vi "校准设置页.vi"() -> ()   [LabVIEW 2016, in "斯坦道CODMn.lvlib"]
uses:
  <vilib>/Analysis/6fits.llb/Curve Fitting Criteria.ctl
  <vilib>/Analysis/NI_AALPro.lvlib
  <vilib>/ptbypt/NI_PtbyPt.lvlib
panel:
  in  "读取公式":bool
  in  "历史数据导入":T1(radio)
  out "校准任务":bool
  in  "二次方程2":cluster{"K":dbl, "B":dbl, "x^2":dbl} {"x^2" format="%#.6g"; "K" format="%#.6g"; "B" format="%#.6g"}
  in  "公式切换阈值滴定数(0~9999)":dbl
  out "校准状态":T2(ring)
  out "模型刷新":bool
  in  "校准按钮":T1(radio)
  in  "校准导入":bool
  in  "曲线模型":T3={"标液浓度1"=0.0, "测量吸光度1"=0.0, "样品1启用"=FALSE, "标液浓度2"=0.0, "测量吸光度2"=0.0, "样品2启用"=FALSE, "标液浓度3"=0.0, "测量吸光度3"=0.0, "样品3启用"=FALSE, "标液浓度4"=0.0, "测量吸光度4"=0.0, "样品4启用"=FALSE, "标液浓度5"=0.0, "测量吸光度5"=0.0, "样品5启用"=FALSE, "模型"=enum."线性", "精度"=4.0, "XY图"=[], "拟合公式"="", "r^2"=0.0, "标样一校准时间"=timestamp(0 s since 1904-01-01), "标样二校准时间"=timestamp(0 s since 1904-01-01), "标样三校准时间"=timestamp(0 s since 1904-01-01), "标样四校准时间"=timestamp(0 s since 1904-01-01), "标样五校准时间"=timestamp(0 s since 1904-01-01), "二次方程"={"K"=0.0, "B"=0.0, "x^2"=0.0}, "标定时间"=timestamp(0 s since 1904-01-01), "拟合公式 2"="", "r^2 2"=0.0} {"r^2 2" format="%.7f"; "标定时间" format="%<%Y/%m/%d %H:%M:%S>T"; "二次方程"."x^2" format="%#.6g"; "二次方程"."K" format="%#.6g"; "二次方程"."B" format="%#.6g"; "标样五校准时间" format="%<%Y/%m/%d %H:%M:%S>T"; "标样四校准时间" format="%<%Y/%m/%d %H:%M:%S>T"; "标样三校准时间" format="%<%Y/%m/%d %H:%M:%S>T"; "标样二校准时间" format="%<%Y/%m/%d %H:%M:%S>T"; "标样一校准时间" format="%<%Y/%m/%d %H:%M:%S>T"; "r^2" format="%.7f"; "测量吸光度5" format="%#.6f"; "测量吸光度4" format="%#.6f"; "测量吸光度3" format="%#.6f"; "测量吸光度2" format="%#.6f"; "测量吸光度1" format="%#.6f"}
  in  "测量模式":T4(ring)
  in  "参数下拉列表":u16(ring) items=["CODMn"=21]
  in  "量程下拉列表":enum16{"低量程", "高量程"}(ring)
  # "校准时间"
  # "标液浓度"
  # "滴定数"
  # "标液一"
  # "标液二"
  # "标液三"
  # "零点"
  # "跨度"
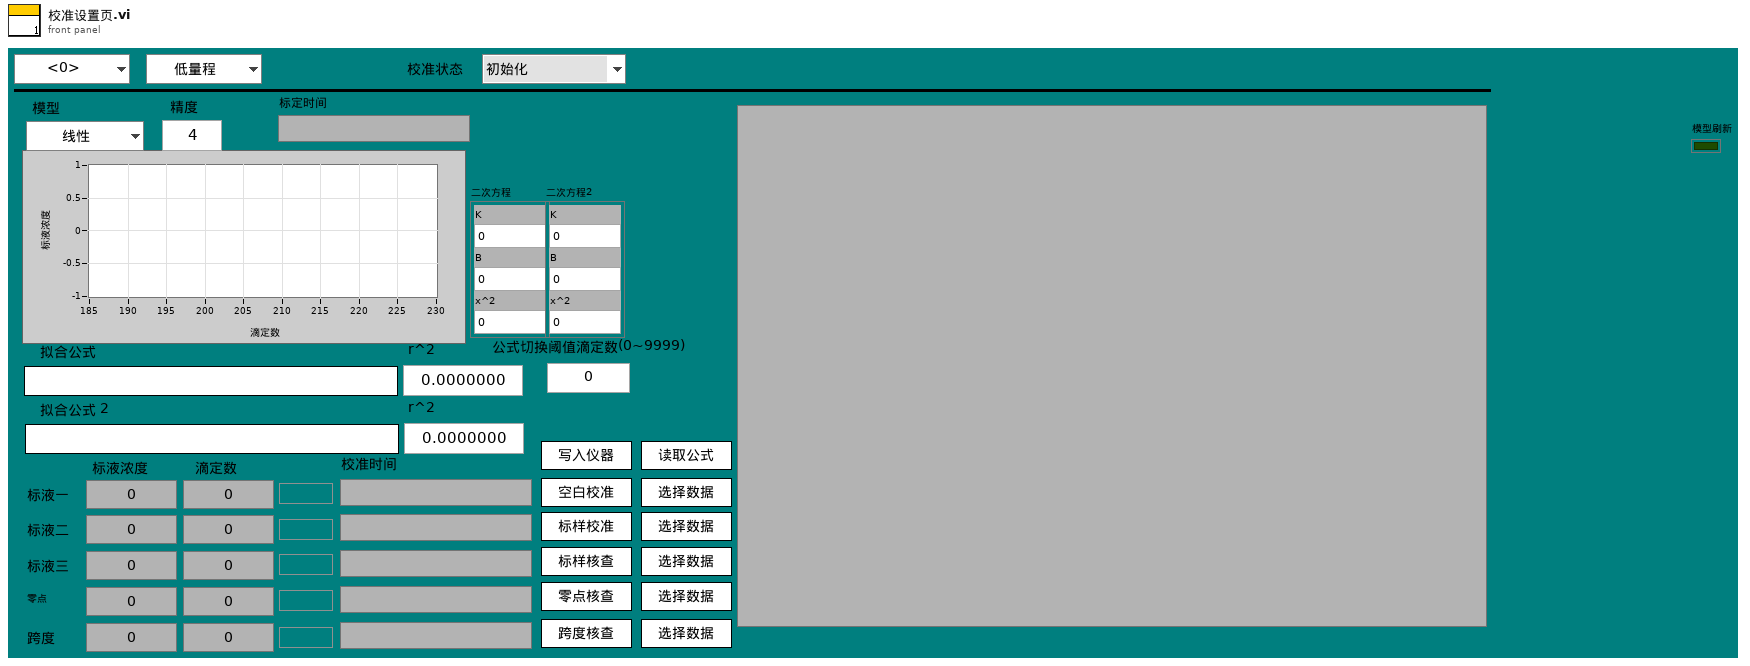
[diagram p1: front panel]
types:
  T1 = enum32{"未选择", "空白校准", "标样校准", "标样核查", "零点核查", "跨度核查"}
  T2 = enum16{"初始化", "解析数据", "判断任务类型", "执行测试任务", "等待测试任务完成", "获取测试数据", "任务结束判定", "计算公式", "结束"}
  T3 = cluster{"标液浓度1":dbl, "测量吸光度1":dbl, "样品1启用":bool, "标液浓度2":dbl, "测量吸光度2":dbl, "样品2启用":bool, "标液浓度3":dbl, "测量吸光度3":dbl, "样品3启用":bool, "标液浓度4":dbl, "测量吸光度4":dbl, "样品4启用":bool, "标液浓度5":dbl, "测量吸光度5":dbl, "样品5启用":bool, "模型":enum32{"线性", "多项式", "折线"}, "精度":dbl, "XY图":cluster{"X Values":dbl[], "Y Values":dbl[]}[], "拟合公式":string, "r^2":dbl, "标样一校准时间":timestamp, "标样二校准时间":timestamp, "标样三校准时间":timestamp, "标样四校准时间":timestamp, "标样五校准时间":timestamp, "二次方程":cluster{"K":dbl, "B":dbl, "x^2":dbl}, "标定时间":timestamp, "拟合公式 2":string, "r^2 2":dbl}
  T4 = enum16{"", "水样测量", "标样核查", "零点核查", "跨度核查", "空白测试", "平行样测试", "加标回收", "空白校准", "标样校准"}
  T5 = typedef "斯坦道CODMn.lvlib/校准任务.ctl" = cluster{"id":u16, "任务类型":enum16{"未选择", "空白校准", "标样校准", "标样核查", "零点核查", "跨度核查"}, "量程下拉列表":enum16{"低量程", "高量程"}, "状态":enum16{"已执行", "待执行", "执行中", "停止"}, "标液浓度":dbl, "吸光值":dbl, "校准时间":timestamp, "报警状态":enum16{"正常数据", "报警数据"}}
  T6 = cluster{"数组 2[0]":sgl, "数组 2[1]":sgl, "数组 2[2]":sgl, "数组 2[3]":sgl, "数组 2[4]":sgl, "数组 2[5]":sgl, "数组 2[6]":sgl, "数组 2[7]":sgl, "数组 2[8]":sgl, "数组 2[9]":sgl, "数组 2[10]":sgl, "数组 2[11]":sgl, "数组 2[12]":sgl, "数组 2[13]":sgl, "数组 2[14]":sgl, "数组 2[15]":sgl, "数组 2[16]":sgl, "数组 2[17]":sgl, "数组 2[18]":sgl, "数组 2[19]":sgl, "数组 2[20]":sgl, "数组 2[21]":sgl, "数组 2[22]":sgl, "数组 2[23]":sgl, "数组 2[24]":sgl, "数组 2[25]":sgl, "数组 2[26]":sgl, "数组 2[27]":sgl, "数组 2[28]":sgl, "数组 2[29]":sgl, "数组 2[30]":sgl, "数组 2[31]":sgl, "数组 2[32]":sgl, "数组 2[33]":sgl, "数组 2[34]":sgl, "数组 2[35]":sgl, "数组 2[36]":sgl, "数组 2[37]":sgl, "数组 2[38]":sgl, "数组 2[39]":sgl, "数组 2[40]":sgl, "数组 2[41]":sgl}
  T7 = cluster{"标液浓度1":dbl, "测量吸光度1":dbl, "样品1启用":bool, "标液浓度2":dbl, "测量吸光度2":dbl, "样品2启用":bool, "标液浓度3":dbl, "测量吸光度3":dbl, "样品3启用":bool, "标液浓度4":dbl, "测量吸光度4":dbl, "样品4启用":bool, "标液浓度5":dbl, "测量吸光度5":dbl, "样品5启用":bool, "模型":enum32{"线性", "多项式", "折线"}, "精度":dbl, "XY图":cluster{"X Values":dbl[], "Y Values":dbl[]}[], "拟合公式":string, "r^2":dbl, "标样一校准时间":timestamp, "标样二校准时间":timestamp, "标样三校准时间":timestamp, "标样四校准时间":timestamp, "标样五校准时间":timestamp, "二次方程":cluster{"c":dbl, "x":dbl, "x^2":dbl}, "标定时间":timestamp, "拟合公式 2":string, "r^2 2":dbl}[][]
  T8 = cluster{"标液浓度1":dbl, "测量吸光度1":dbl, "样品1启用":bool, "标液浓度2":dbl, "测量吸光度2":dbl, "样品2启用":bool, "标液浓度3":dbl, "测量吸光度3":dbl, "样品3启用":bool, "标液浓度4":dbl, "测量吸光度4":dbl, "样品4启用":bool, "标液浓度5":dbl, "测量吸光度5":dbl, "样品5启用":bool, "模型":enum32{"线性", "多项式", "折线"}, "精度":dbl, "XY图":cluster{"X Values":dbl[], "Y Values":dbl[]}[], "拟合公式":string, "r^2":dbl, "标样一校准时间":timestamp, "标样二校准时间":timestamp, "标样三校准时间":timestamp, "标样四校准时间":timestamp, "标样五校准时间":timestamp, "二次方程":cluster{"c":dbl, "x":dbl, "x^2":dbl}, "标定时间":timestamp, "拟合公式 2":string, "r^2 2":dbl}
  T9 = typedef "NI_AALPro.lvlib/Curve Fitting Criteria.ctl" = u16
  T10 = enum32{"Bad", "Idle", "Run top level", "Running"}
  T11 = cluster{"时间":timestamp, "标液值":dbl, "检测值":dbl, "吸光值":dbl}
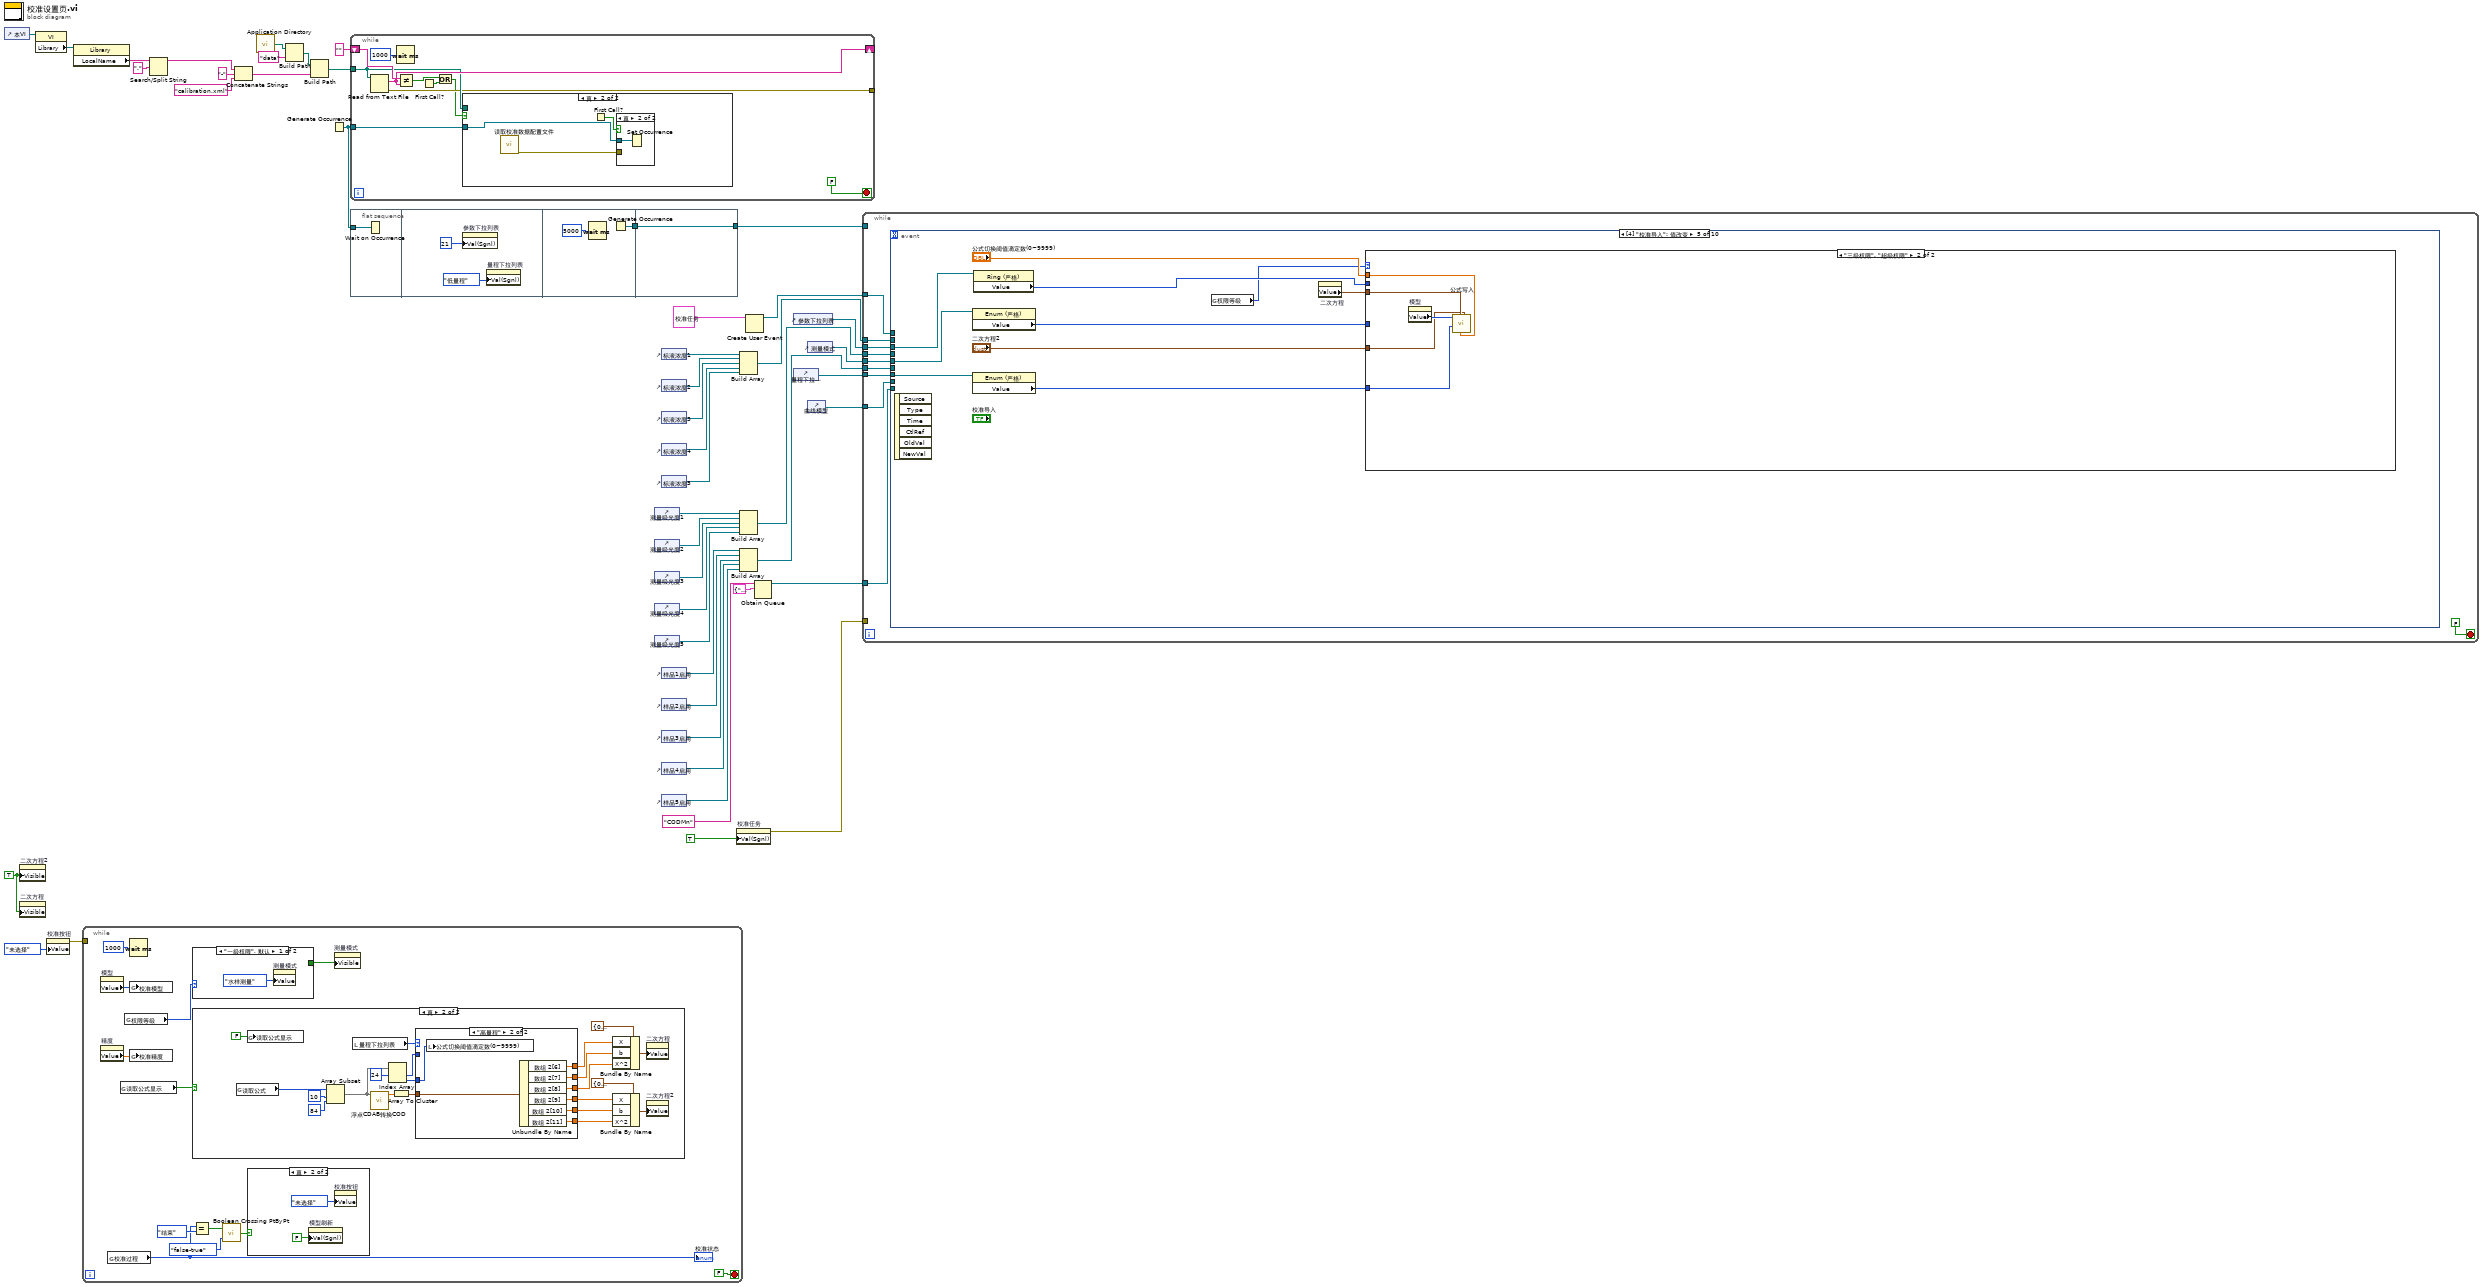
[diagram p0: block diagram]
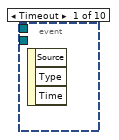
[diagram p4: hidden frame]
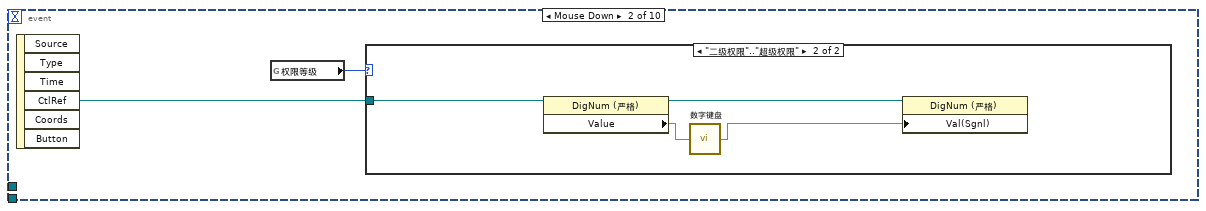
[diagram p5: hidden frame]
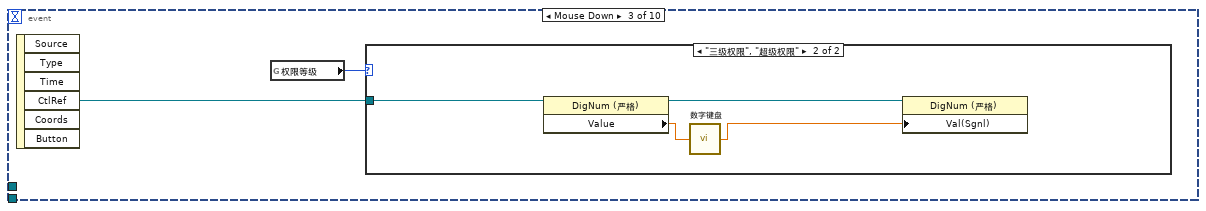
[diagram p7: hidden frame]
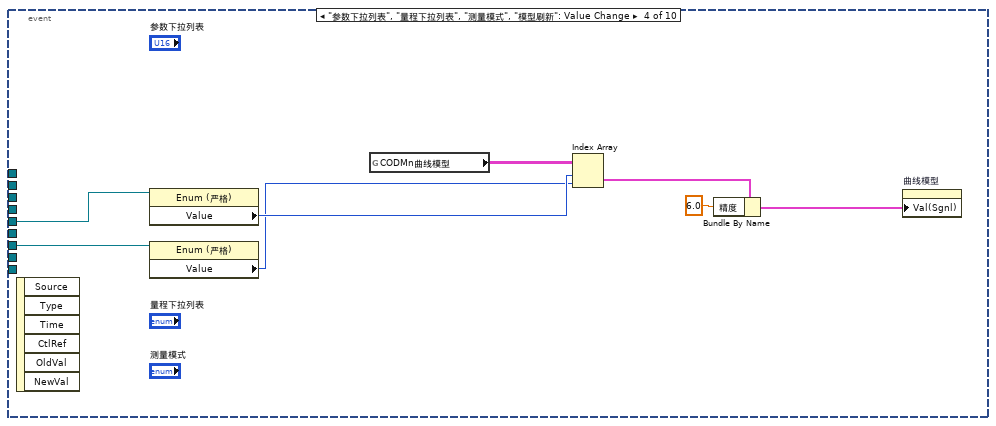
[diagram p9: hidden frame]
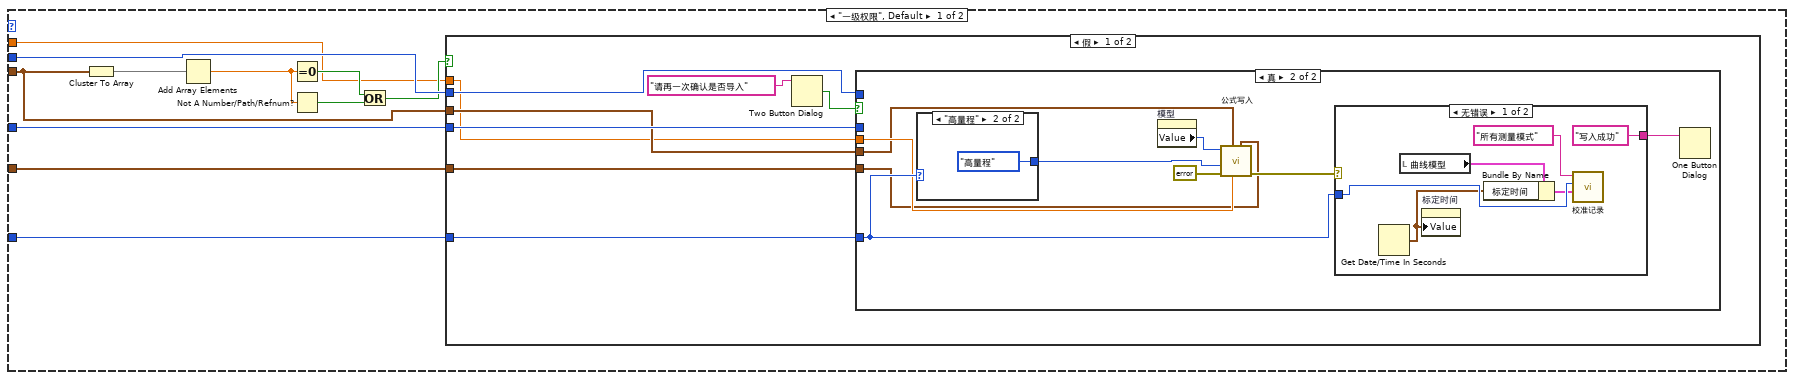
[diagram p10: hidden frame]
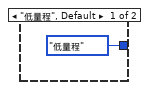
[diagram p12: hidden frame]
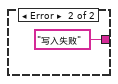
[diagram p13: hidden frame]
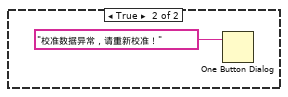
[diagram p14: hidden frame]
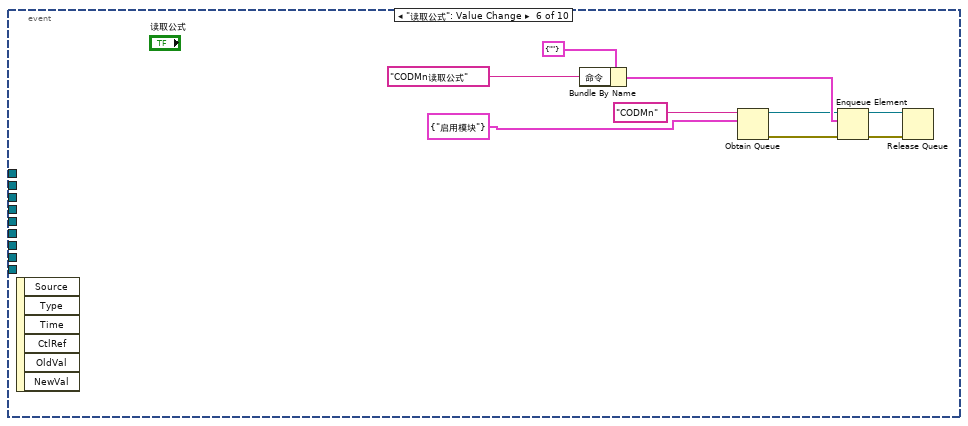
[diagram p15: hidden frame]
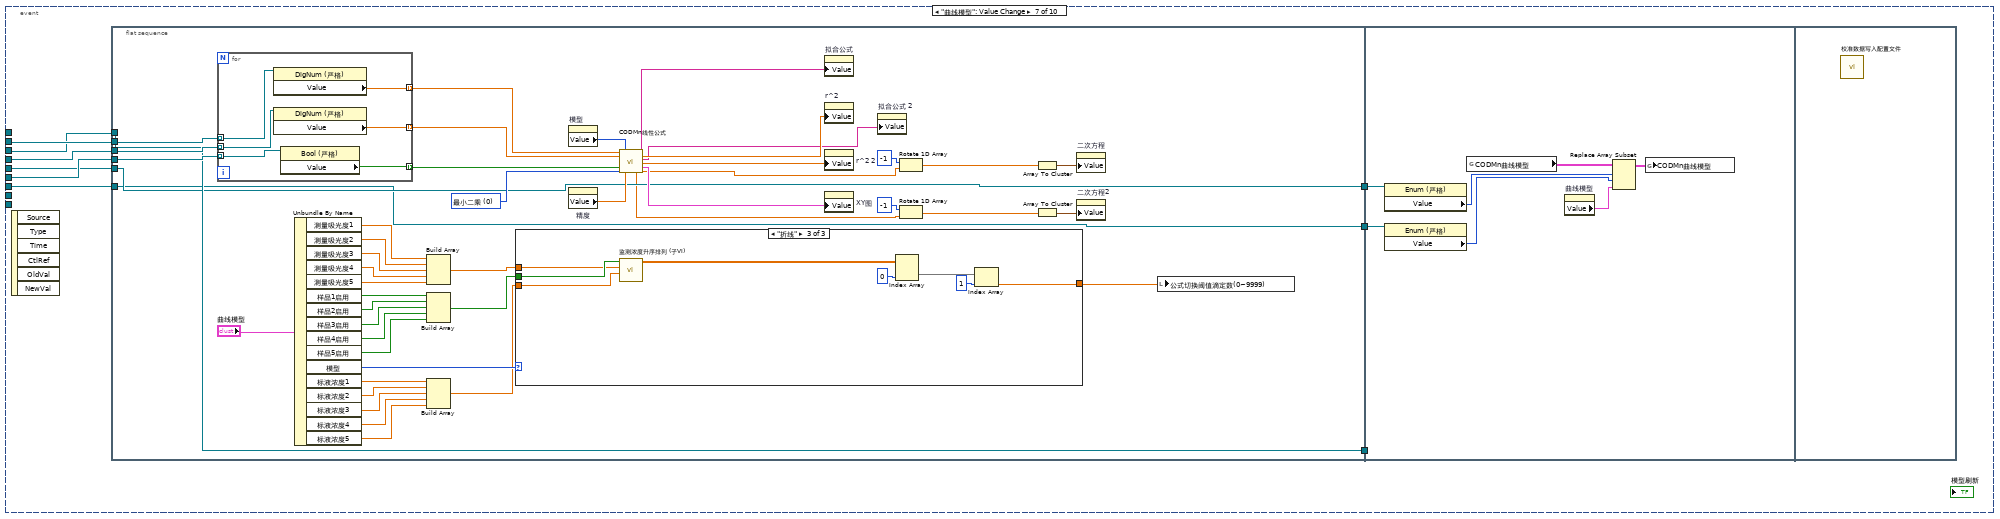
[diagram p16: hidden frame]
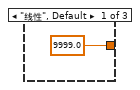
[diagram p17: hidden frame]
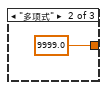
[diagram p18: hidden frame]
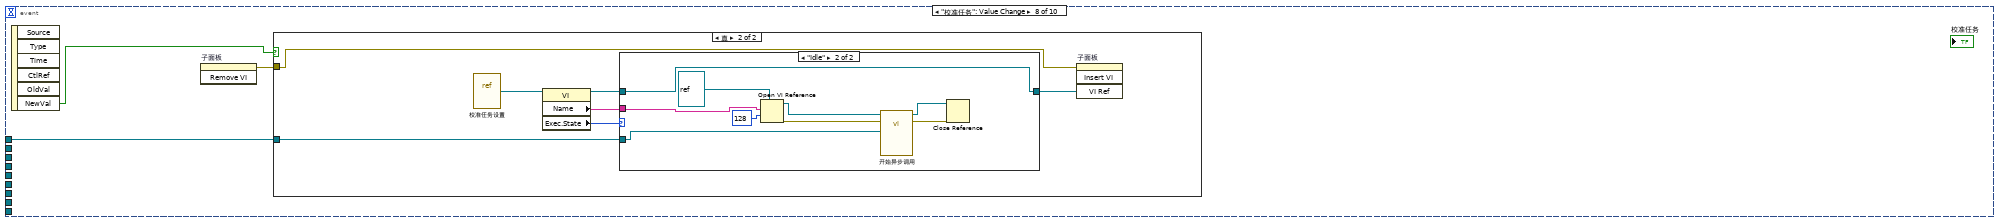
[diagram p19: hidden frame]
diagram:
  w2 = TRUE ("可见")
  n1 = control-ref of="本VI"() -> (w9:refnum<vi>)
  n2 = property on="二次方程2" class="Clust (严格)"("Visible"=w2) -> ()  [unwired: 2 in, 2 out]
  n3 = property on="二次方程" class="Clust (严格)"("Visible"=w2) -> ()  [unwired: 2 in, 2 out]
  n4 = property class="VI"(reference=w9) -> ("Library"=w18:refnum<vi>)  [unwired: 1 in, 2 out]
  n5 = property on="校准按钮" class="RadioBtnsControl (严格)"("Value"=T1."未选择" ("校准按钮")) -> (error out=w1:errorcluster)  [unwired: 2 in, 1 out]
  n6 = property class="Library"(reference=w18) -> ("LocalName"=w16:string)  [unwired: 1 in, 2 out]
  n7 = while {
    tunnel: w1 -> [_]
    stop <- FALSE stop-if-true
    n8 = property on="模型" class="Enum (严格)"() -> ("Value"=w52:enum32{"线性", "多项式", "折线"})  [unwired: 2 in, 2 out]
    n9 = property on="精度" class="DigNum (严格)"() -> ("Value"=w51:dbl)  [unwired: 2 in, 2 out]
    n10 = global read "校准数据全局变量.vi" "校准过程"() -> (w53:T2)
    "校准状态" <- w53
    n11 = global read "COD内部交互全局.vi" "读取公式显示"() -> (w49:bool)
    n12 = global read "CODMN外部API.vi" "权限等级"() -> (w50:enum16{"一级权限", "二级权限", "三级权限", "超级权限"})
    n13 = Wait (ms)(milliseconds to wait=u32 1000 ("等待时间（毫秒）")) -> ()  [unwired: 1 out]
    n14 = global write "校准数据全局变量.vi" "校准模型"(w52) -> ()
    n15 = global write "校准数据全局变量.vi" "校准精度"(w51) -> ()
    n16 = case shown="\"一级权限\", 默认" w50 {
      tunnel: [_ TRUE ("可见")] -> w58
      frame "一级权限", Default {
        n17 = property on="测量模式" class="Enum (严格)"("Value"=T4."水样测量" ("测量模式")) -> ()  [unwired: 2 in, 2 out]
      }
      frame "三级权限", "超级权限" {
      }
    }
    n18 = case shown="真" w49 {
      frame False {
      }
      frame True {
        n19 = global read "COD内部交互全局.vi" "读取公式"() -> (w75:u16[])
        n20 = global write "COD内部交互全局.vi" "读取公式显示"(FALSE ("读取公式显示")) -> ()
        n21 = Array Subset(array=w75, index=10 ("索引"), length=84 ("长度")) -> (w77:u16[])
        n22 = local read "量程下拉列表"() -> (w74:enum16{"低量程", "高量程"})
        n23 = call "浮点CDAB转换COD.vi"("数组"=w77) -> ("数组 2"=w80:sgl[])  [unwired: 10 in]
        n24 = Index Array(array=w77, index #1=24 ("索引")) -> (element #1=w71:u16, element #2=w72:u16)  [unwired: 1 in]
        n25 = Array To Cluster(array=w80) -> (cluster=w73:T6)
        n26 = case shown="\"高量程\"" w74 {
          tunnel: w73 -> [w89 w96]
          tunnel: w72 -> [_ w97]
          tunnel: w71 -> [w88 _]
          tunnel: [w87 w95] -> w68
          tunnel: [w86 w94] -> w67
          tunnel: [w85 w93] -> w66
          tunnel: [w84 w92] -> w65
          tunnel: [w83 w91] -> w64
          tunnel: [w82 w90] -> w63
          frame "低量程", Default {
            n27 = local write "公式切换阈值滴定数(0~9999)"(w88) -> ()
            n28 = Unbundle By Name(w89) -> ("数组 2[0]"=w87:sgl, "数组 2[1]"=w86:sgl, "数组 2[2]"=w85:sgl, "数组 2[3]"=w84:sgl, "数组 2[4]"=w83:sgl, "数组 2[5]"=w82:sgl)
          }
          frame "高量程" {
            n29 = local write "公式切换阈值滴定数(0~9999)"(w97) -> ()
            n30 = Unbundle By Name(w96) -> ("数组 2[6]"=w95:sgl, "数组 2[7]"=w94:sgl, "数组 2[8]"=w93:sgl, "数组 2[9]"=w92:sgl, "数组 2[10]"=w91:sgl, "数组 2[11]"=w90:sgl)
          }
        }
        n31 = Bundle By Name(cluster=cluster{"X":dbl, "b":dbl, "X^2":dbl} {"X"=0.0, "b"=0.0, "X^2"=0.0} ("方程系数"), "X"=w68, "b"=w67, "X^2"=w66) -> (w62:cluster{"X":dbl, "b":dbl, "X^2":dbl})
        n32 = Bundle By Name(cluster=cluster{"X":dbl, "b":dbl, "X^2":dbl} {"X"=0.0, "b"=0.0, "X^2"=0.0} ("方程系数"), "X"=w65, "b"=w64, "X^2"=w63) -> (w61:cluster{"X":dbl, "b":dbl, "X^2":dbl})
        n33 = property on="二次方程" class="Clust (严格)"("Value"=w62) -> ()  [unwired: 2 in, 2 out]
        n34 = property on="二次方程2" class="Clust (严格)"("Value"=w61) -> ()  [unwired: 2 in, 2 out]
      }
    }
    n35 = Equal?(x=w53, y=T2."结束" ("校准过程")) -> (x = y?=w57:bool)
    n36 = call <vilib>:"Boolean Crossing PtByPt.vi"("direction"=enum16{"either", "false-true", "true-false"}."false-true", "input"=w57) -> ("crossing"=w55:bool)  [unwired: 1 in]
    n37 = case shown="真" w55 {
      frame False {
      }
      frame True {
        n38 = property on="模型刷新" class="Bool (严格)"("Val(Sgnl)"=FALSE ("值(信号)")) -> ()  [unwired: 2 in, 2 out]
        n39 = property on="校准按钮" class="RadioBtnsControl (严格)"("Value"=T1."未选择" ("校准按钮")) -> ()  [unwired: 2 in, 2 out]
      }
    }
    n40 = property on="测量模式" class="Enum (严格)"("Visible"=w58) -> ()  [unwired: 2 in, 2 out]
  }
  n41 = Search/Split String(string=w16, search string/char (-)="." ("搜索字符串/字符(-)")) -> (substring before match=w14:string)  [unwired: 1 in, 2 out]
  n42 = Concatenate Strings(w14, "-" ("字符串"), "calibration.xml" ("名称或相对路径")) -> (w11:string)
  n43 = call <vilib>:"Application Directory.vi"() -> ("Application Directory"=w19:path)
  n44 = Build Path(base path=w19, name or relative path="data" ("名称或相对路径")) -> (appended path=w17:path)
  n45 = Build Path(base path=w17, name or relative path=w11) -> (appended path=w10:path)
  n46 = Generate Occurrence() -> (w7:refnum<k4>)
  n47 = while {
    shift-right: [w109] -> _
    shift-left: "" -> [w110]
    tunnel: w10 -> [w108]
    tunnel: [w106] -> _
    tunnel: w7 -> [w102]
    stop <- FALSE stop-if-true
    n48 = Read from Text File(file (use dialog)=w108) -> (text=w109:string, error out=w106:errorcluster)  [unwired: 3 in, 2 out]
    n49 = Wait (ms)(milliseconds to wait=u32 1000 ("等待时间（毫秒）")) -> ()  [unwired: 1 out]
    n50 = Not Equal?(x=w110, y=w109) -> (x != y?=w104:bool)
    n51 = First Call?() -> (First Call?: T/F=w105:bool)
    n52 = Or(x=w104, y=w105) -> (x .or. y?=w103:bool)
    n53 = case shown="真" w103 {
      tunnel: w108 -> [_ _]
      tunnel: w102 -> [_ w113]
      frame False {
      }
      frame True {
        n54 = call "读取校准数据配置文件.vi"() -> ("错误输出"=w112:errorcluster)  [unwired: 11 in]
        n55 = First Call?() -> (First Call?: T/F=w114:bool)
        n56 = case shown="真" w114 {
          tunnel: w113 -> [_ w115]
          tunnel: w112 -> [_ _]
          frame False {
          }
          frame True {
            n57 = Set Occurrence(w115) -> ()
          }
        }
      }
    }
  }
  n58 = flat-sequence {
    tunnel: w7 -> [w116]
    tunnel: [w120] -> w48
    tunnel: [w121] -> w47
    tunnel: w48 -> [w121]
    frame #0 {
      n59 = Wait on Occurrence(2:w116) -> ()  [unwired: 2 in, 1 out]
    }
    frame #1 {
      n60 = property on="参数下拉列表" class="Ring (严格)"("Val(Sgnl)"=u16 21 ("值(信号)")) -> ()  [unwired: 2 in, 2 out]
      n61 = property on="量程下拉列表" class="Enum (严格)"("Val(Sgnl)"=enum16{"低量程", "高量程"}."低量程" ("值(信号)")) -> ()  [unwired: 2 in, 2 out]
    }
    frame #2 {
      n62 = Wait (ms)(milliseconds to wait=u32 5000 ("等待时间（毫秒）")) -> ()  [unwired: 1 out]
      n63 = Generate Occurrence() -> (w120:refnum<k4>)
    }
    frame #3 {
    }
  }
  n64 = control-ref of="测量吸光度1"() -> (w35:refnum<vi>)
  n65 = control-ref of="测量吸光度2"() -> (w36:refnum<vi>)
  n66 = control-ref of="测量吸光度3"() -> (w37:refnum<vi>)
  n67 = control-ref of="测量吸光度4"() -> (w38:refnum<vi>)
  n68 = control-ref of="测量吸光度5"() -> (w39:refnum<vi>)
  n69 = control-ref of="标液浓度1"() -> (w33:refnum<vi>)
  n70 = control-ref of="标液浓度2"() -> (w32:refnum<vi>)
  n71 = control-ref of="标液浓度3"() -> (w31:refnum<vi>)
  n72 = control-ref of="标液浓度4"() -> (w30:refnum<vi>)
  n73 = control-ref of="标液浓度5"() -> (w29:refnum<vi>)
  n74 = control-ref of="样品1启用"() -> (w45:refnum<vi>)
  n75 = control-ref of="样品2启用"() -> (w44:refnum<vi>)
  n76 = control-ref of="样品3启用"() -> (w43:refnum<vi>)
  n77 = control-ref of="样品4启用"() -> (w42:refnum<vi>)
  n78 = control-ref of="样品5启用"() -> (w41:refnum<vi>)
  n79 = property on="校准任务" class="Bool (严格)"("Val(Sgnl)"=TRUE ("值(信号)")) -> (error out=w5:errorcluster)  [unwired: 2 in, 1 out]
  n80 = Build Array(w33, w32, w31, w30, w29) -> (w28:refnum<vi>[])
  n81 = Build Array(w35, w36, w37, w38, w39) -> (w34:refnum<vi>[])
  n82 = Build Array(w45, w44, w43, w42, w41) -> (w40:refnum<vi>[])
  n83 = Create User Event(user event datatype=T5 {"id"=0, "任务类型"=enum."未选择", "量程下拉列表"=enum."低量程", "状态"=enum."已执行", "标液浓度"=0.0, "吸光值"=0.0, "校准时间"=timestamp(0 s since 1904-01-01), "报警状态"=enum."正常数据"} ("校准任务")) -> (user event=w3:refnum<user-event>)  [unwired: 1 in, 1 out]
  n84 = Obtain Queue(name (unnamed)="CODMn" ("名称（未命名）"), element data type=cluster{"命令":string, "data":variant} {"命令"="", "data"=variant}) -> (queue out=w24:refnum<queue>)  [unwired: 3 in, 2 out]
  n85 = control-ref of="参数下拉列表"() -> (w46:refnum<vi>)
  n86 = control-ref of="量程下拉列表"() -> (w26:refnum<vi>)
  n87 = control-ref of="测量模式"() -> (w27:refnum<vi>)
  n88 = control-ref of="曲线模型"() -> (w21:refnum<vi>)
  n89 = while {
    tunnel: w47 -> [_]
    tunnel: w46 -> [w130]
    tunnel: w40 -> [w129]
    tunnel: w34 -> [w128]
    tunnel: w28 -> [w127]
    tunnel: w27 -> [w126]
    tunnel: w26 -> [w125]
    tunnel: w24 -> [w124]
    tunnel: w21 -> [w123]
    tunnel: w5 -> [_]
    tunnel: w3 -> [w122]
    stop <- FALSE stop-if-true
    n90 = event shown="[4] \"校准导入\": 值改变" {
      selector: _ -> [_ _ _ _ _ _ _ _ _ _]
      dyn-events: _ -> [_ _ _ _ _ _ _ _ _ _]
      timeout: _ -> [_ _ _ _ _ _ _ _ _ _]
      tunnel: w130 -> [_ _ _ _ w161 _ w218 _ w320 w348]
      tunnel: w129 -> [_ _ _ _ _ _ w222 _ _ _]
      tunnel: w128 -> [_ _ _ _ _ _ w221 _ _ _]
      tunnel: w127 -> [_ _ _ _ _ _ w220 _ _ _]
      tunnel: w126 -> [_ _ _ w151 w159 _ w216 _ w315 w343]
      tunnel: w125 -> [_ _ _ w150 w157 _ w214 _ w319 w347]
      tunnel: w124 -> [_ _ _ _ _ _ _ _ w321 w349]
      tunnel: w123 -> [_ _ _ _ _ _ _ _ w313 _]
      tunnel: w122 -> [_ _ _ _ _ _ _ w293 w312 w342]
      event Timeout {
        n91 = event-data() -> ()  [unwired: 1 in, 3 out]
      }
      event "曲线模型.标液浓度1", "曲线模型.标液浓度2", "曲线模型.标液浓度3", "曲线模型.标液浓度4", "曲线模型.标液浓度5", "曲线模型.精度": Mouse Down {
        n92 = event-data() -> ("CtlRef"=w133:refnum<vi>)  [unwired: 1 in, 5 out]
        n93 = global read "CODMN外部API.vi" "权限等级"() -> (w132:enum16{"一级权限", "二级权限", "三级权限", "超级权限"})
        n94 = case shown="\"二级权限\"..\"超级权限\"" w132 {
          tunnel: w133 -> [_ w137]
          frame "一级权限", Default {
          }
          frame "二级权限".."超级权限" {
            n95 = property class="DigNum (严格)"(reference=w137) -> (reference out=w135:refnum<vi>, "Value"=w136:dbl)  [unwired: 1 in, 1 out]
            n96 = call "数字键盘.vi"("OldNumber"=w136) -> ("NewNumber"=w134:sgl)
            n97 = property class="DigNum (严格)"(reference=w135, "Val(Sgnl)"=w134) -> ()  [unwired: 1 in, 2 out]
          }
        }
      }
      event "曲线模型.测量吸光度1", "曲线模型.测量吸光度2", "曲线模型.测量吸光度3", "曲线模型.测量吸光度4", "曲线模型.测量吸光度5": Mouse Down {
        n98 = event-data() -> ("CtlRef"=w139:refnum<vi>)  [unwired: 1 in, 5 out]
        n99 = global read "CODMN外部API.vi" "权限等级"() -> (w138:enum16{"一级权限", "二级权限", "三级权限", "超级权限"})
        n100 = case shown="\"三级权限\", \"超级权限\"" w138 {
          tunnel: w139 -> [_ w143]
          frame "一级权限", Default {
          }
          frame "三级权限", "超级权限" {
            n101 = property class="DigNum (严格)"(reference=w143) -> (reference out=w141:refnum<vi>, "Value"=w142:dbl)  [unwired: 1 in, 1 out]
            n102 = call "数字键盘.vi"("OldNumber"=w142) -> ("NewNumber"=w140:sgl)
            n103 = property class="DigNum (严格)"(reference=w141, "Val(Sgnl)"=w140) -> ()  [unwired: 1 in, 2 out]
          }
        }
      }
      event "参数下拉列表", "量程下拉列表", "测量模式", "模型刷新": Value Change {
        n104 = event-data() -> ()  [unwired: 1 in, 6 out]
        n105 = property class="Enum (严格)"(reference=w151) -> ("Value"=w148:T4)  [unwired: 1 in, 2 out]
        n106 = property class="Enum (严格)"(reference=w150) -> ("Value"=w147:enum16{"低量程", "高量程"})  [unwired: 1 in, 2 out]
        n107 = global read "校准数据全局变量.vi" "CODMn曲线模型"() -> (w149:T7)
        n108 = Index Array(array=w149, index (row)=w148, index (col)=w147) -> (element=w146:T8)
        n109 = Bundle By Name(cluster=w146, "精度"=6.0 ("值")) -> (w145:T8)
        n110 = property on="曲线模型" class="Clust (严格)"("Val(Sgnl)"=w145) -> ()  [unwired: 2 in, 2 out]
      }
      event "校准导入": Value Change {
        n111 = event-data() -> ()  [unwired: 1 in, 6 out]
        n112 = property class="Enum (严格)"(reference=w159) -> ("Value"=w158:T4)  [unwired: 1 in, 2 out]
        n113 = property class="Enum (严格)"(reference=w157) -> ("Value"=w156:enum16{"低量程", "高量程"})  [unwired: 1 in, 2 out]
        n114 = property class="Ring (严格)"(reference=w161) -> ("Value"=w160:u16)  [unwired: 1 in, 2 out]
        n115 = global read "CODMN外部API.vi" "权限等级"() -> (w153:enum16{"一级权限", "二级权限", "三级权限", "超级权限"})
        n116 = property on="二次方程" class="Clust (严格)"() -> ("Value"=w152:cluster{"K":dbl, "B":dbl, "x^2":dbl})  [unwired: 2 in, 2 out]
        n117 = case shown="\"三级权限\", \"超级权限\"" w153 {
          tunnel: w160 -> [w172 _]
          tunnel: w158 -> [w171 _]
          tunnel: w156 -> [w170 w203]
          tunnel: w152 -> [w164 w201]
          tunnel: "公式切换阈值滴定数(0~9999)" -> [w163 w202]
          tunnel: "二次方程2" -> [w162 w200]
          frame "一级权限", Default {
            n118 = Cluster To Array(cluster=w164) -> (array=w169:dbl[])
            n119 = Add Array Elements(numeric array=w169) -> (sum=w168:dbl)
            n120 = Equal To 0?(x=w168) -> (x = 0?=w166:bool)
            n121 = Not A Number/Path/Refnum?(number/path/refnum=w168) -> (NaN/Path/Refnum?=w167:bool)
            n122 = Or(x=w166, y=w167) -> (x .or. y?=w165:bool)
            n123 = case shown="假" w165 {
              tunnel: w172 -> [w180 _]
              tunnel: w171 -> [w179 _]
              tunnel: w170 -> [w178 _]
              tunnel: w164 -> [w175 _]
              tunnel: w163 -> [w174 _]
              tunnel: w162 -> [w173 _]
              frame False {
                n124 = Two Button Dialog(message="请再一次确认是否导入" ("消息")) -> (T button?=w176:bool)  [unwired: 2 in]
                n125 = case shown="真" w176 {
                  tunnel: w180 -> [_ _]
                  tunnel: w179 -> [_ _]
                  tunnel: w178 -> [_ w188]
                  tunnel: w175 -> [_ w181]
                  tunnel: w174 -> [_ w184]
                  tunnel: w173 -> [_ w182]
                  frame False {
                  }
                  frame True {
                    n126 = case shown="\"高量程\"" w188 {
                      tunnel: [enum16{"低量程", "高量程"}."低量程" ("量程选择") enum16{"低量程", "高量程"}."高量程" ("量程选择")] -> w185
                      frame "低量程", Default {
                      }
                      frame "高量程" {
                      }
                    }
                    n127 = property on="模型" class="Enum (严格)"() -> ("Value"=w183:enum32{"线性", "多项式", "折线"})  [unwired: 2 in, 2 out]
                    n128 = call "公式写入.vi"("公式 2"=w182, "公式切换阈值滴定数(0-9999)"=w184, "公式"=w181, "Error in"=errorcluster {"status"=FALSE, "code"=0, "source"=""} ("error out"), "量程选择"=w185, "模型"=w183) -> ("error out"=w187:errorcluster)  [unwired: 5 in]
                    n129 = case shown="无错误" w187 {
                      tunnel: ["写入成功" "写入失败"] -> w189
                      tunnel: w188 -> [w196 _]
                      frame No Error {
                        n130 = Get Date/Time In Seconds() -> (seconds since 1Jan1904=w193:timestamp)
                        n131 = local read "曲线模型"() -> (w194:T3)
                        n132 = property on="标定时间" class="AbsTime (严格)"("Value"=w193) -> ()  [unwired: 2 in, 2 out]
                        n133 = Bundle By Name(cluster=w194, "标定时间"=w193) -> (w192:T3)
                        n134 = call "校准记录.vi"("曲线模型"=w192, "量程"=w196, "测量模式"="所有测量模式") -> ()  [unwired: 8 in, 1 out]
                      }
                      frame Error {
                      }
                    }
                    n135 = One Button Dialog(message=w189) -> ()  [unwired: 1 in, 1 out]
                  }
                }
              }
              frame True {
                n136 = One Button Dialog(message="校准数据异常，请重新校准！" ("消息")) -> ()  [unwired: 1 in, 1 out]
              }
            }
          }
          frame "三级权限", "超级权限" {
            n137 = property on="模型" class="Enum (严格)"() -> ("Value"=w204:enum32{"线性", "多项式", "折线"})  [unwired: 2 in, 2 out]
            n138 = call "公式写入.vi"("公式 2"=w200, "公式切换阈值滴定数(0-9999)"=w202, "公式"=w201, "量程选择"=w203, "模型"=w204) -> ()  [unwired: 6 in, 1 out]
          }
        }
      }
      event "读取公式": Value Change {
        n139 = event-data() -> ()  [unwired: 1 in, 6 out]
        n140 = Bundle By Name(cluster=cluster{"命令":string} {"命令"=""} ("元素"), "命令"="CODMn读取公式" ("名称（未命名）")) -> (w211:cluster{"命令":string})
        n141 = Obtain Queue(name (unnamed)="CODMn" ("名称（未命名）"), element data type=cluster{"命令":string} {"命令"="启用模块"} ("元素")) -> (queue out=w207:refnum<queue>, error out=w208:errorcluster)  [unwired: 3 in, 1 out]
        n142 = Enqueue Element(queue=w207, element=w211, error in (no error)=w208) -> (queue out=w206:refnum<queue>, error out=w205:errorcluster)  [unwired: 1 in, 1 out]
        n143 = Release Queue(queue=w206, error in (no error)=w205) -> ()  [unwired: 1 in, 3 out]
      }
      event "曲线模型": Value Change {
        n144 = event-data() -> ()  [unwired: 1 in, 6 out]
        n145 = flat-sequence {
          tunnel: w222 -> [w268]
          tunnel: w221 -> [w266]
          tunnel: w220 -> [w264]
          tunnel: [w256] -> w219
          tunnel: w218 -> [w256]
          tunnel: [w255] -> w217
          tunnel: w216 -> [w255]
          tunnel: [w254] -> w215
          tunnel: w214 -> [w254]
          tunnel: w219 -> [_]
          tunnel: w217 -> [w290]
          tunnel: w215 -> [w289]
          frame #0 {
            w260 = T9 0 items=["最小二乘", "最小绝对残差", "Bisquare"] ("method")
            n146 = for {
              tunnel: w268 -> [w284] mode=indexing
              tunnel: [w283] -> w267 mode=indexing
              tunnel: w266 -> [w282] mode=indexing
              tunnel: [w281] -> w265 mode=indexing
              tunnel: w264 -> [w280] mode=indexing
              tunnel: [w279] -> w263 mode=indexing
              n147 = property class="DigNum (严格)"(reference=w280) -> ("Value"=w279:dbl)  [unwired: 1 in, 2 out]
              n148 = property class="DigNum (严格)"(reference=w282) -> ("Value"=w281:dbl)  [unwired: 1 in, 2 out]
              n149 = property class="Bool (严格)"(reference=w284) -> ("Value"=w283:bool)  [unwired: 1 in, 2 out]
            }
            n150 = Unbundle By Name("曲线模型") -> ("测量吸光度1"=w252:dbl, "测量吸光度2"=w251:dbl, "测量吸光度3"=w250:dbl, "测量吸光度4"=w248:dbl, "测量吸光度5"=w249:dbl, "样品1启用"=w247:bool, "样品2启用"=w246:bool, "样品3启用"=w245:bool, "样品4启用"=w244:bool, "样品5启用"=w243:bool, "模型"=w237:enum32{"线性", "多项式", "折线"}, "标液浓度1"=w236:dbl, "标液浓度2"=w235:dbl, "标液浓度3"=w234:dbl, "标液浓度4"=w233:dbl, "标液浓度5"=w232:dbl)
            n151 = Build Array(w252, w251, w250, w248, w249) -> (w241:dbl[])
            n152 = Build Array(w247, w246, w245, w244, w243) -> (w242:bool[])
            n153 = Build Array(w236, w235, w234, w233, w232) -> (w231:dbl[])
            n154 = case shown="\"折线\"" w237 {
              tunnel: w242 -> [_ _ w276]
              tunnel: w241 -> [_ _ w275]
              tunnel: [9999.0 ("数值") 9999.0 ("数值") w277] -> w238
              tunnel: w231 -> [_ _ w274]
              frame "线性", Default {
              }
              frame "多项式" {
              }
              frame "折线" {
                n155 = call "监测浓度升序排列 (子VI).vi"("标液浓度"=w274, "滴定数"=w275, "启用"=w276) -> ("输出数组"=w273:dbl[][])  [unwired: 8 in]
                n156 = Index Array(array=w273, index (col)=0 ("禁用的索引 (列)")) -> (element=w271:dbl[])  [unwired: 1 in]
                n157 = Index Array(array=w271, index=1 ("索引")) -> (element=w277:dbl)
              }
            }
            n158 = property on="模型" class="Enum (严格)"() -> ("Value"=w262:enum32{"线性", "多项式", "折线"})  [unwired: 2 in, 2 out]
            n159 = property on="精度" class="DigNum (严格)"() -> ("Value"=w261:dbl)  [unwired: 2 in, 2 out]
            n160 = call "CODMn线性公式.vi"("标液浓度"=w263, "滴定数"=w265, "启用"=w267, "method"=w260, "模型"=w262, "精度"=w261) -> ("Polynomial Coefficients 2"=w228:dbl[], "拟合方程"=w259:string, "r^2"=w258:dbl, "拟合方程 2"=w240:string, "r^2 2"=w239:dbl, "XY图"=w257:cluster{"X Values":dbl[], "Y Values":dbl[]}[], "Polynomial Coefficients"=w224:dbl[])  [unwired: 7 in]
            n161 = property on="拟合公式" class="Str"("Value"=w259) -> ()  [unwired: 2 in, 2 out]
            n162 = property on="r^2" class="DigNum (严格)"("Value"=w258) -> ()  [unwired: 2 in, 2 out]
            n163 = property on="r^2 2" class="DigNum (严格)"("Value"=w239) -> ()  [unwired: 2 in, 2 out]
            n164 = property on="XY图" class="XYGraph (严格)"("Value"=w257) -> ()  [unwired: 2 in, 2 out]
            n165 = property on="拟合公式 2" class="Str"("Value"=w240) -> ()  [unwired: 2 in, 2 out]
            n166 = Rotate 1D Array(1:w224, 2:-1 ("n")) -> (0:w226:dbl[])
            n167 = Rotate 1D Array(1:w228, 2:-1 ("n")) -> (0:w230:dbl[])
            n168 = Array To Cluster(array=w226) -> (cluster=w223:cluster{"[0]":dbl, "[1]":dbl, "[2]":dbl})
            n169 = Array To Cluster(array=w230) -> (cluster=w227:cluster{"[0]":dbl, "[1]":dbl, "[2]":dbl})
            n170 = property on="二次方程" class="Clust (严格)"("Value"=w223) -> ()  [unwired: 2 in, 2 out]
            n171 = property on="二次方程2" class="Clust (严格)"("Value"=w227) -> ()  [unwired: 2 in, 2 out]
            n172 = local write "公式切换阈值滴定数(0~9999)"(w238) -> ()
          }
          frame #1 {
            n173 = property class="Enum (严格)"(reference=w290) -> ("Value"=w287:T4)  [unwired: 1 in, 2 out]
            n174 = property class="Enum (严格)"(reference=w289) -> ("Value"=w288:enum16{"低量程", "高量程"})  [unwired: 1 in, 2 out]
            n175 = global read "校准数据全局变量.vi" "CODMn曲线模型"() -> (w286:T7)
            n176 = property on="曲线模型" class="Clust (严格)"() -> ("Value"=w291:T3)  [unwired: 2 in, 2 out]
            n177 = Replace Array Subset(array=w286, new element=w291, index (row)=w287, index (col)=w288) -> (w285:T7)
            n178 = global write "校准数据全局变量.vi" "CODMn曲线模型"(w285) -> ()
          }
          frame #2 {
            n179 = call "校准数据写入配置文件.vi"() -> ()  [unwired: 11 in, 1 out]
          }
        }
      }
      event "校准任务": Value Change {
        n180 = event-data() -> ("NewVal"=w294:bool)  [unwired: 1 in, 5 out]
        n181 = invoke on="子面板" class="SubPnl" method="Remove VI"() -> (error out=w292:errorcluster)  [unwired: 3 in, 2 out]
        n182 = case shown="真" w294 {
          tunnel: w293 -> [_ w298]
          tunnel: w292 -> [_ w295]
          frame False {
          }
          frame True {
            n183 = vi-ref "校准任务设置.vi"() -> (w301:refnum<vi>)
            n184 = property class="VI"(reference=w301) -> (reference out=w297:refnum<vi>, "Name"=w299:string, "Exec.State"=w300:T10)  [unwired: 1 in, 1 out]
            n185 = case shown="\"Idle\"" w300 {
              tunnel: w299 -> [_ w311]
              tunnel: w298 -> [_ w306]
              tunnel: w297 -> [w302 w303]
              tunnel: [w302 w303] -> w296
              frame "Bad", Default {
              }
              frame "Idle" {
                n186 = Open VI Reference(type specifier VI Refnum (for type only)=refnum<vi> refnum ("类型说明符VI引用句柄（仅用于类型）"), vi path=w311, options=128 ("选项")) -> (vi reference=w308:refnum<vi>, error out=w307:errorcluster)  [unwired: 3 in]
                n187 = call-by-ref "开始异步调用"(reference=w308, error in=w307, "用户事件"=w306) -> (reference out=w305:refnum<vi>, error out=w304:errorcluster)  [unwired: 11 in]
                n188 = Close Reference(reference=w305, error in (no error)=w304) -> ()  [unwired: 1 out]
              }
            }
            n189 = invoke on="子面板" class="SubPnl" method="Insert VI"(error in=w295, "VI Ref"=w296) -> ()  [unwired: 2 in, 4 out]
          }
        }
      }
      event "校准按钮": Value Change {
        n190 = event-data() -> ("CtlRef"=w314:refnum<vi>, "NewVal"=w316:T1)  [unwired: 1 in, 4 out]
        n191 = Not Equal?(x=w316, y=T1."未选择") -> (x != y?=w317:bool)
        n192 = case shown="真" w317 {
          tunnel: w321 -> [_ _]
          tunnel: w320 -> [_ w329]
          tunnel: w319 -> [_ w327]
          tunnel: w316 -> [_ w331]
          tunnel: w315 -> [_ _]
          tunnel: w314 -> [_ _]
          tunnel: w313 -> [_ _]
          tunnel: w312 -> [_ w330]
          frame False {
          }
          frame True {
            (unwired) u16 21 items=["CODMn"=21] ("参数下拉列表")
            n193 = property class="Enum (严格)"(reference=w327) -> ("Value"=w326:enum16{"低量程", "高量程"})  [unwired: 1 in, 2 out]
            n194 = property class="Ring (严格)"(reference=w329) -> ("Value"=w328:u16)  [unwired: 1 in, 2 out]
            n195 = local read "曲线模型"() -> (w324:T3)
            n196 = case shown="\"跨度核查\"" w331 {
              tunnel: w324 -> [_ w333 w335 w336 w338 w340]
              tunnel: [_ w332 w334 w337 w339 w341] -> w323
              frame "未选择", Default {
              }
              frame "空白校准" {
                n197 = Unbundle By Name(w333) -> ("标液浓度1"=w332:dbl)
              }
              frame "标样校准" {
                n198 = Unbundle By Name(w335) -> ("标液浓度2"=w334:dbl)
              }
              frame "标样核查" {
                n199 = Unbundle By Name(w336) -> ("标液浓度3"=w337:dbl)
              }
              frame "零点核查" {
                n200 = Unbundle By Name(w338) -> ("标液浓度4"=w339:dbl)
              }
              frame "跨度核查" {
                n201 = Unbundle By Name(w340) -> ("标液浓度5"=w341:dbl)
              }
            }
            n202 = Bundle By Name(cluster=T5 {"id"=0, "任务类型"=enum."未选择", "量程下拉列表"=enum."低量程", "状态"=enum."待执行", "标液浓度"=0.0, "吸光值"=0.0, "校准时间"=timestamp(0 s since 1904-01-01), "报警状态"=enum."正常数据"} ("校准任务"), "id"=w328, "任务类型"=w331, "量程下拉列表"=w326, "标液浓度"=w323) -> (w325:T5)
            n203 = Generate User Event(user event=w330, event data cluster=w325) -> ()  [unwired: 2 in, 2 out]
          }
        }
      }
      event "历史数据导入": Value Change {
        n204 = event-data() -> ("NewVal"=w344:T1)  [unwired: 1 in, 5 out]
        n205 = Not Equal?(x=w344, y=T1."未选择") -> (x != y?=w345:bool)
        n206 = case shown="真" w345 {
          tunnel: w349 -> [_ _]
          tunnel: w348 -> [_ w359]
          tunnel: w347 -> [_ w358]
          tunnel: w344 -> [_ w352]
          tunnel: w343 -> [_ _]
          tunnel: w342 -> [_ w356]
          frame False {
          }
          frame True {
            n207 = property class="Enum (严格)"(reference=w358) -> ("Value"=w354:enum16{"低量程", "高量程"})  [unwired: 1 in, 2 out]
            n208 = property class="Ring (严格)"(reference=w359) -> ("Value"=w355:u16)  [unwired: 1 in, 2 out]
            n209 = property on="历史数据导入" class="RadioBtnsControl (严格)"("Value"=T1."未选择" ("历史数据导入")) -> ()  [unwired: 2 in, 2 out]
            n210 = call "校准数据选择表.vi"("历史数据导入"=w352, "量程下拉列表"=w354, "table"="CODMn") -> ("布尔"=w357:bool, "输出"=w350:T11)  [unwired: 7 in]
            n211 = case shown="真" w357 {
              tunnel: w350 -> [_ w365]
              tunnel: w356 -> [_ w369]
              tunnel: w355 -> [_ w366]
              tunnel: w354 -> [_ w364]
              tunnel: w352 -> [_ w363]
              frame False {
              }
              frame True {
                n212 = Unbundle By Name(w365) -> ("标液值"=w362:dbl, "吸光值"=w361:dbl, "时间"=w360:timestamp)
                n213 = Bundle By Name(cluster=T5 {"id"=0, "任务类型"=enum."未选择", "量程下拉列表"=enum."低量程", "状态"=enum."已执行", "标液浓度"=0.0, "吸光值"=0.0, "校准时间"=timestamp(0 s since 1904-01-01), "报警状态"=enum."正常数据"} ("事件数据"), "id"=w366, "任务类型"=w363, "量程下拉列表"=w364, "标液浓度"=w362, "吸光值"=w361, "校准时间"=w360) -> (w367:T5)
                n214 = Generate User Event(user event=w369, event data cluster=w367) -> ()  [unwired: 2 in, 2 out]
              }
            }
          }
        }
      }
    }
  }
